vi "Write State_.vi"(10 "State:":T1=enum."FaultState", 11 "TestDataLog in":refnum<class "TestDataLog.lvclass">) -> (3 "TestDataLog out":refnum<class "TestDataLog.lvclass">)   [LabVIEW 2013, in "TestDataLog.lvclass"]
uses:
  TestDataLog.lvclass
  Typedefs/StateSelector.ctl
  TestDataLog.lvclass/TestDataLog.ctl
  Typedefs/ILCBTTypedefs.lvlib
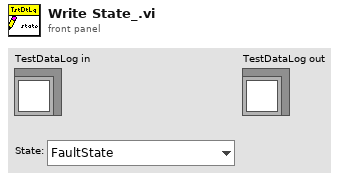
[diagram p1: front panel]
types:
  T1 = typedef "ILCBTTypedefs.lvlib/StateSelector.ctl" = enum16{"EnabledState", "FaultState", "OffState", "StandbyState"}
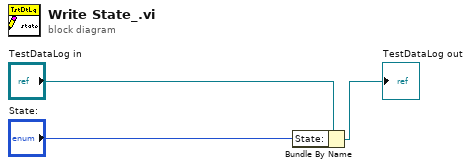
[diagram p0: block diagram]
diagram:
  n1 = Bundle By Name(cluster="TestDataLog in", "State:"="State:") -> (→"TestDataLog out":refnum<class "TestDataLog.lvclass">)
